vi "Check_Recipe.vi"(0 "Step In":i32, 5 "Number of Steps":i32, 7 "Time Remaining":dbl, 9 "Display In":string, 11 "error in (no error)":errorcluster) -> (4 "Step Out":i32, 6 "State":T1=enum."Staged", 10 "Display Out":string, 15 "error out":errorcluster)   [LabVIEW 2026]
uses:
  controls/System_Status.ctl
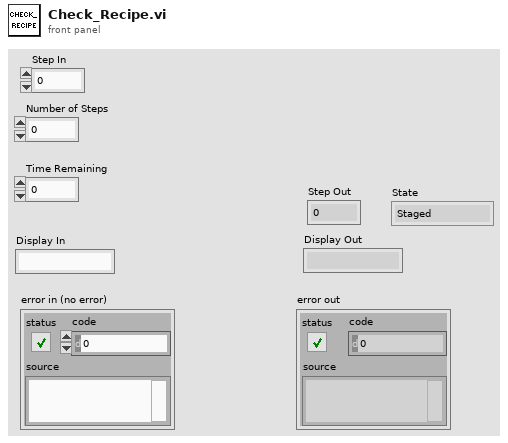
[diagram p1: front panel]
types:
  T1 = typedef "System_Status.ctl" = enum16{"Idle", "Staged", "Cooking", "Paused", "Buzzer Alert"}
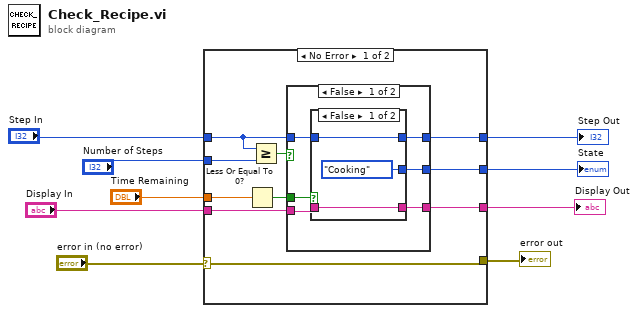
[diagram p0: block diagram]
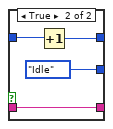
[diagram p2: hidden frame]
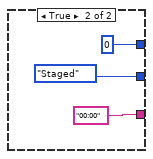
[diagram p3: hidden frame]
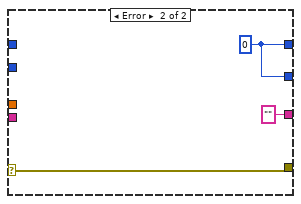
[diagram p4: hidden frame]
diagram:
  n1 = case shown="No Error" "error in (no error)" {
    selector: "error in (no error)" -> [w10 w36]
    tunnel: "Step In" -> [w19 _]
    tunnel: "Number of Steps" -> [w18 _]
    tunnel: "Display In" -> [w17 _]
    tunnel: [w16 "" ("Display In")] -> w6
    tunnel: "Time Remaining" -> [w15 _]
    tunnel: [w14 w38] -> w4
    tunnel: [w13 w38] -> w3
    tunnel: [w10 w36] -> w1
    frame No Error {
      n2 = Less Or Equal To 0?(x=w15) -> (x <= 0?=w12:bool)
      n3 = Greater Or Equal?(x=w19, y=w18) -> (x >= y?=w11:bool)
      n4 = case shown="False" w11 {
        tunnel: w12 -> [w25 _]
        tunnel: w19 -> [w24 _]
        tunnel: [w23 0] -> w13
        tunnel: [w22 System_Status."Staged" ("State")] -> w14
        tunnel: [w20 "00:00"] -> w16
        tunnel: w17 -> [w21 _]
        frame False {
          n5 = case shown="False" w25 {
            tunnel: [w27 w30] -> w23
            tunnel: w24 -> [w27 w31]
            tunnel: [System_Status."Cooking" ("State") System_Status."Idle" ("State")] -> w22
            tunnel: w21 -> [w26 w29]
            tunnel: [w26 w29] -> w20
            frame False {
            }
            frame True {
              n6 = Increment(x=w31) -> (x+1=w30:i32)
            }
          }
        }
        frame True {
        }
      }
    }
    frame Error {
      w38 = 0 ("Step In")
    }
  }
  "Display Out" <- w6
  "State" <- w4
  "Step Out" <- w3
  "error out" <- w1
